vi "Dt_Marker.vi"(7 "ROI Descriptor":T2 {"Contours"."Type" items=["No Selection", "Point", "Line", "Rectangle", "Oval", "Polygon", "Freehand Region", "Annulus", "Unused2", "Unused3", "Broken Line", "Freehand Line", "Rotated Rectangle"]}, 8 "Minimum Match Score":sgl=400.0 min=0 max=1000 format="%.2f", 9 "PrevCnt":cluster{"x":sgl, "y":sgl}, 10 "Img_Mrk":T1, 11 "Img_Mod":T1) -> (0 "GlobalRect_Matches":sgl[](array[numeric]), 1 "Position":cluster{"x":sgl, "y":sgl}, 2 "RefCnt":cluster{"Left":sgl, "Top":sgl}, 3 "Img_Mod_Out":T1, 5 "x = 0?":bool)   [LabVIEW 2013]
uses:
  <vilib>/vision/Image Controls.llb/IMAQ Image.ctl
  <vilib>/Utility/error.llb/DialogType.ctl
  <vilib>/vision/NI_Vision_Development_Module.lvlib
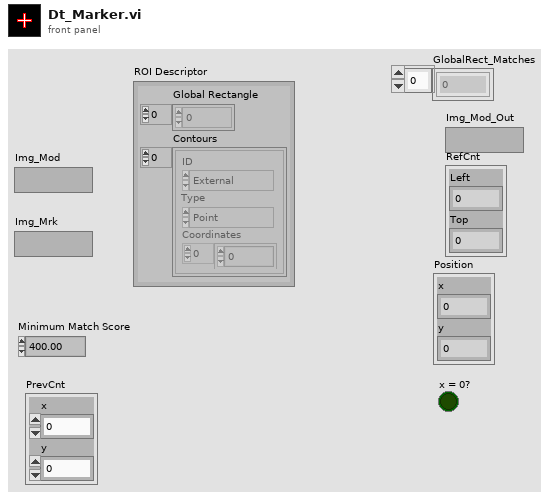
[diagram p1: front panel]
types:
  T1 = typedef "IMAQ Image.ctl" = refnum<image>
  T2 = typedef "ROI Descriptor" = cluster{"Global Rectangle":i32[], "Contours":cluster{"ID":enum32{"External", "Internal"}, "Type":u32, "Coordinates":i32[]}[]}
  T3 = typedef "DialogType.ctl" = u16
  T4 = cluster{"Position":cluster{"x":sgl, "y":sgl}, "Angle":sgl, "Scale":sgl, "Score":sgl, "Bounding Box":cluster{"x":sgl, "y":sgl}[]}[]
  T5 = cluster{"Left":sgl, "Top":sgl, "Right":sgl, "Bottom":sgl}
  T6 = cluster{"Position":cluster{"x":sgl, "y":sgl}, "Angle":sgl, "Scale":sgl, "Score":sgl, "Bounding Box":cluster{"x":sgl, "y":sgl}[]}
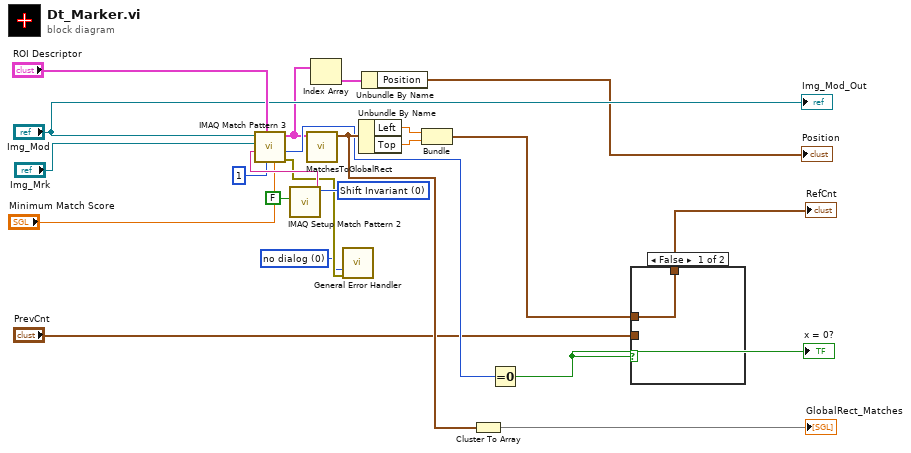
[diagram p0: block diagram]
diagram:
  w9 = T3 0 items=["no dialog", "OK message", "continue or stop message", "OK message + warnings", "continue/stop + warnings"] ("type of dialog (OK msg:1)")
  w21 = u16 0 items=["Shift Invariant", "Rotation Invariant"] ("Match Mode")
  n1 = call "IMAQ Setup Match Pattern 2"("Subpixel Accuracy"=FALSE, "Match Mode"=w21) -> ("Match Pattern Setup Data"=w22:string)  [unwired: 3 in, 6 out]
  n2 = call "IMAQ Match Pattern 3"("Minimum Match Score"="Minimum Match Score", "Number of Matches Requested"=1, "ROI Descriptor"="ROI Descriptor", "Match Pattern Setup Data"=w22, "Template Image"="Img_Mrk", "Image"="Img_Mod") -> ("error out"=w10:errorcluster, "Number of Matches"=w7:i32, "Matches"=w3:T4)  [unwired: 1 in, 2 out]
  n3 = call "MatchesToGlobalRect.vi"("Matches"=w3) -> ("Global Rectangle"=w13:T5)  [unwired: 10 in]
  n4 = Index Array(array=w3) -> (element=w2:T6)  [unwired: 1 in]
  n5 = call <vilib>:"General Error Handler.vi"("type of dialog (OK msg:1)"=w9, "error in (no error)"=w10) -> ()  [unwired: 9 in, 5 out]
  n6 = Unbundle By Name(w13) -> ("Left"=w15:sgl, "Top"=w16:sgl)
  n7 = Unbundle By Name(w2) -> ("Position"=→"Position":cluster{"x":sgl, "y":sgl})
  n8 = Bundle("Left"=w15, "Top"=w16) -> (w4:cluster{"Left":sgl, "Top":sgl})  [unwired: 1 in]
  n9 = Cluster To Array(cluster=w13) -> (array=→"GlobalRect_Matches":sgl[])
  n10 = Equal To 0?(x=w7) -> (x = 0?=w8:bool)
  "x = 0?" <- w8
  n11 = case shown="False" w8 {
    tunnel: [w23 w24] -> w5
    tunnel: "PrevCnt" -> [_ w24]
    tunnel: w4 -> [w23 _]
    frame False {
    }
    frame True {
    }
  }
  "RefCnt" <- w5
  "Img_Mod_Out" <- "Img_Mod"
